vi "Post-Build Action.vi"(5 "Files Generated by Build":path[](array[path]), 6 "Top Level/Always Included VIs":path[](array[path]), 7 "Destination Path":path, 8 "error in (no error)":errorcluster, 9 "Target Name":string, 10 "Build Specification Name":string, 11 "Project Path":path) -> (0 "error out":errorcluster)   [LabVIEW 2020]
uses:
  <vilib>/Utility/error.llb/Error Cluster From Error Code.vi
  <vilib>/regexp/Match Regular Expression.xnode
  <vilib>/ErrorRing/Error Ring.xnode
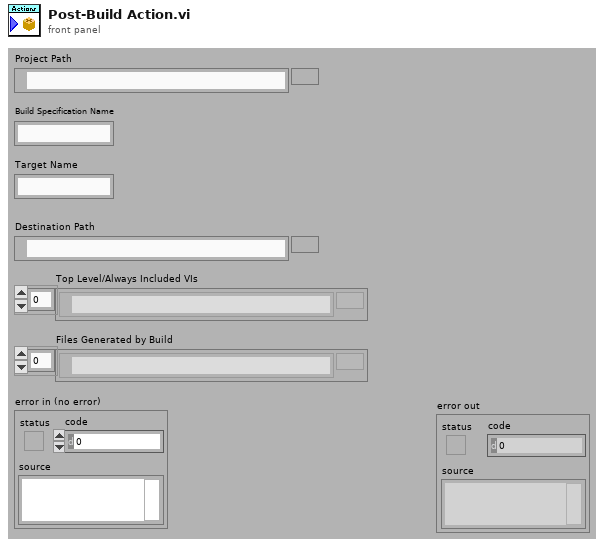
[diagram p1: front panel]
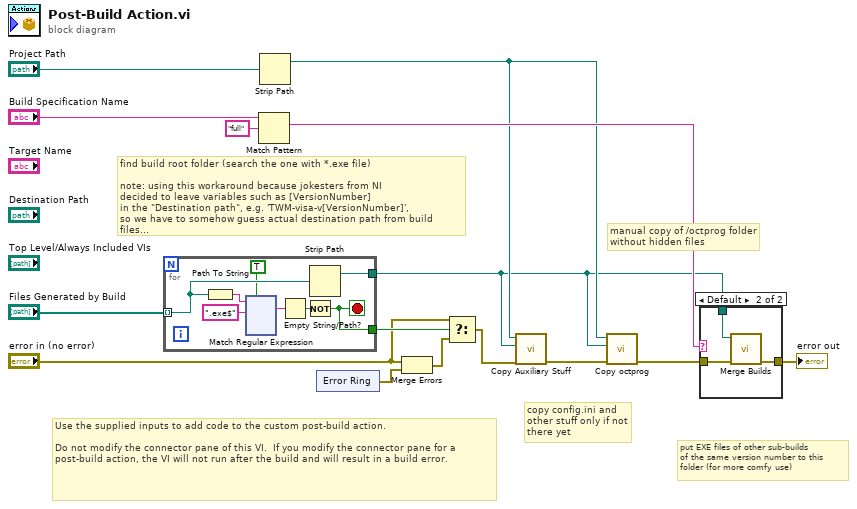
[diagram p0: block diagram]
diagram:
  # "copy config.ini and\nother stuff only if not\nthere yet"
  # "put EXE files of other sub-builds\nof the same version number to this\nfolder (for more comfy use)"
  # "find build root folder (search the one with *.exe file)\n\nnote: using this workaround because jokesters from NI\ndecided to leave variables such as [VersionNumber]\nin the \"Destination path\", e.g. 'TWM-visa-v[VersionNumber]',\nso we have to somehow guess actual destination path from build files..."
  # "manual copy of /octprog folder\nwithout hidden files"
  # "Use the supplied inputs to add code to the custom post-build action.\n\nDo not modify the connector pane of this VI.  If you modify the connector pane for a post-build action, the VI will not run after the build and will result in a build error."
  n1 = for {
    tunnel: "Files Generated by Build" -> [w20] mode=indexing
    tunnel: [w19] -> w1
    tunnel: [w17] -> w13
    stop <- w17 stop-if-true
    n2 = Path To String(path=w20) -> (string=w22:string)
    n3 = xnode "Match Regular Expression"("input string"=w22, "regular expression"=".exe$", "ignore case? (F)"=TRUE) -> ("whole match"=w21:string)  [unwired: 3 in, 4 out]
    n4 = Empty String/Path?(string/path=w21) -> (empty?=w18:bool)
    n5 = Not(x=w18) -> (.not. x?=w17:bool)
    n6 = Strip Path(path=w20) -> (stripped path=w19:path)  [unwired: 1 out]
  }
  n7 = Match Pattern(string="Build Specification Name", regular expression="full") -> (match substring=w5:string)  [unwired: 1 in, 3 out]
  n8 = Strip Path(path="Project Path") -> (stripped path=w2:path)  [unwired: 1 out]
  n9 = xnode "Error Ring"() -> ("error out"=w14:errorcluster)
  n10 = Merge Errors("error in (no error)", w14) -> (w12:errorcluster)
  n11 = Select(t="error in (no error)", s=w13, f=w12) -> (s? t:f=w3:errorcluster)
  n12 = call "Copy Auxiliary Stuff.vi"("error in"=w3, "Build Destination Folder Path"=w1, "lvProject folder path"=w2) -> ("error out"=w4:errorcluster)  [unwired: 8 in]
  n13 = call "Copy octprog.vi"("error in"=w4, "Destination Path"=w1, "lvProject path"=w2) -> ("error out"=w9:errorcluster)  [unwired: 8 in]
  n14 = case shown="Default" w5 {
    tunnel: w9 -> [w138 w141]
    tunnel: w1 -> [_ w140]
    tunnel: [w138 w139] -> w8
    frame "" {
    }
    frame Default {
      n15 = call "Merge Builds.vi"("error in"=w141, "Destination Path"=w140) -> ("error out"=w139:errorcluster)  [unwired: 9 in]
    }
  }
  "error out" <- w8
